vi "Query Board Resources.vi"(8 "error in (no error)":errorcluster, 11 "board":u32) -> (0 "error out":errorcluster, 1 "found":bool, 3 "board resource":T1)   [LabVIEW 2020, in "AIM664LV.lvlib"]
uses:
  AIM664LV.lvlib
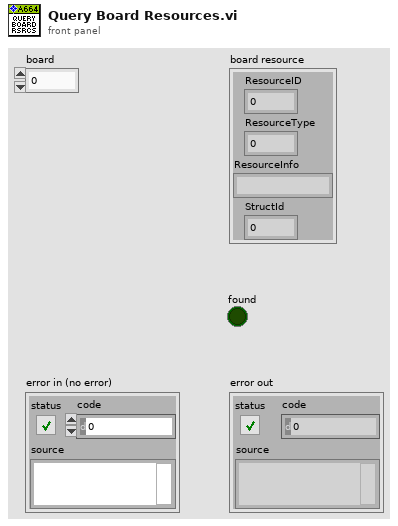
[diagram p1: front panel]
types:
  T1 = cluster{"ResourceID":u32, "ResourceType":u32, "ResourceInfo":string, "StructId":u32}
  T2 = typedef "AIM664LV.lvlib/hwResource_board.ctl" = cluster{"boardId":u32, "ServerResourceInfo":cluster{"ResourceID":u32, "ResourceType":u32, "ResourceInfo":string, "StructId":u32}}
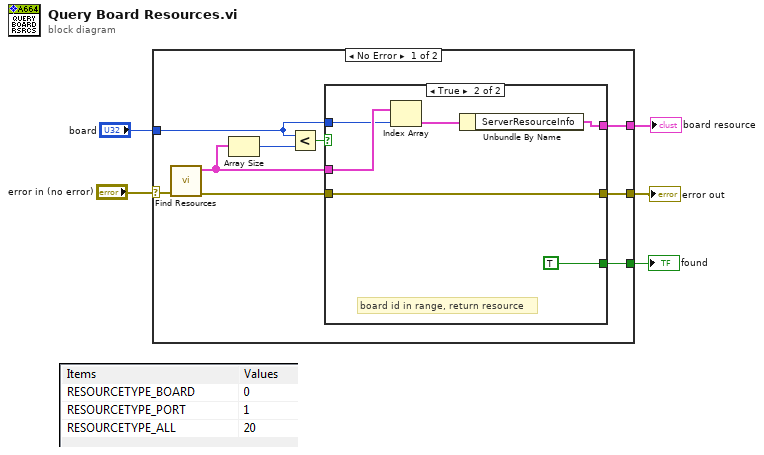
[diagram p0: block diagram]
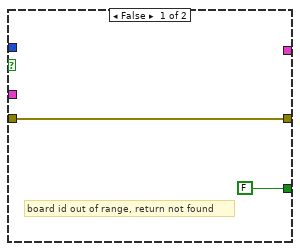
[diagram p2: hidden frame]
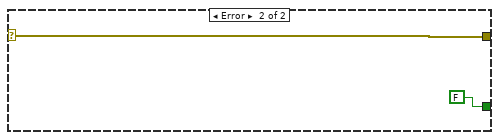
[diagram p3: hidden frame]
diagram:
  n1 = case shown="No Error" "error in (no error)" {
    selector: "error in (no error)" -> [w14 w24]
    tunnel: "board" -> [w9 _]
    tunnel: [w7 w24] -> w3
    tunnel: [w8 _] -> w2
    tunnel: [w6 FALSE ("found")] -> w1
    frame No Error {
      n2 = call "Find Resources.vi"("error in"=w14) -> ("error out"=w12:errorcluster, "Boards"=w11:T2[])  [unwired: 8 in, 1 out]
      n3 = Array Size(array=w11) -> (size(s)=w10:i32)
      n4 = Less?(x=w9, y=w10) -> (x < y?=w13:bool)
      n5 = case shown="True" w13 {
        tunnel: w12 -> [w15 w19]
        tunnel: w11 -> [_ w22]
        tunnel: w9 -> [_ w18]
        tunnel: [_ w20] -> w8
        tunnel: [w15 w19] -> w7
        tunnel: [FALSE TRUE] -> w6
        frame False {
          # "board id out of range, return not found"
        }
        frame True {
          # "board id in range, return resource"
          n6 = Index Array(array=w22, index=w18) -> (element=w21:T2)
          n7 = Unbundle By Name(w21) -> ("ServerResourceInfo"=w20:T1)
        }
      }
    }
    frame Error {
    }
  }
  "error out" <- w3
  "board resource" <- w2
  "found" <- w1
